vi "RXD_gloval.vi"(7 "종료문자열":string="\r\n", 9 "Vesa_Status":T1=enum."Idel", 11 "SERIAL.COM_Port":refnum<visa-resource-name>="COM1") -> (3 "수신문자":string)   [LabVIEW 2014]
uses:
  VESA_Status.ctl
  bus_button.xctl
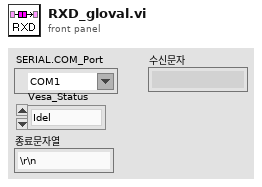
[diagram p1: front panel]
types:
  T1 = typedef "bus_button.xctl/VESA_Status.ctl" = enum16{"Init", "Wait", "Connect", "DisConnect", "Idel", "Exit"}
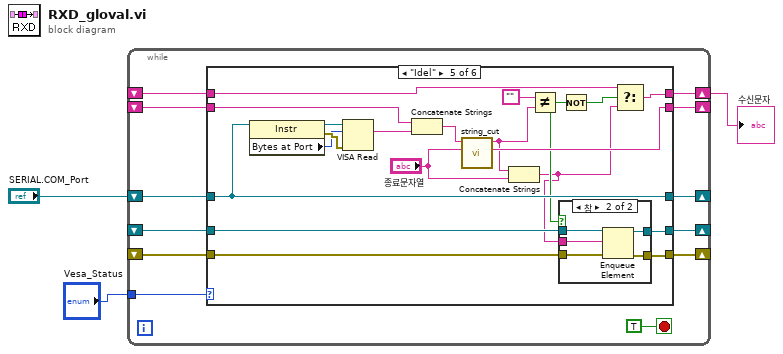
[diagram p0: block diagram]
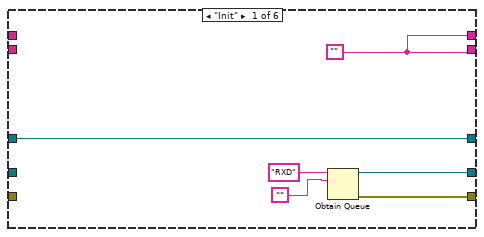
[diagram p2: hidden frame]
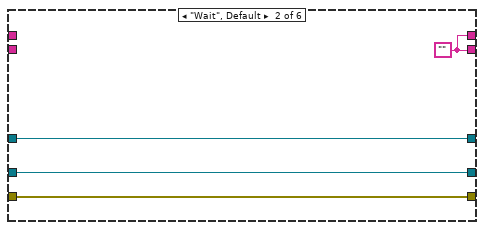
[diagram p3: hidden frame]
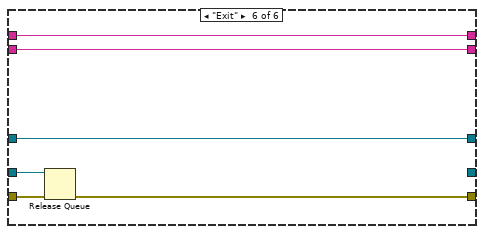
[diagram p7: hidden frame]
diagram:
  n1 = while {
    shift-right: [w14] -> _
    shift-left: _ -> [w10]
    shift-right: [w13] -> _
    shift-left: _ -> [w11]
    shift-right: [w12] -> _
    shift-left: _ -> [w9]
    shift-right: [w7] -> _
    shift-left: "SERIAL.COM_Port" -> [w8]
    tunnel: "Vesa_Status" -> [w6]
    shift-right: [w5] -> w1
    shift-left: _ -> [w4]
    stop <- TRUE stop-if-true
    n2 = case shown="\"Idel\"" w6 {
      tunnel: [w19 w24 w29 w34 w46 _] -> w14
      tunnel: [w18 w25 w30 w35 w47 w64] -> w13
      tunnel: [w16 w22 w28 w33 w43 w68] -> w12
      tunnel: w11 -> [_ w25 w30 w35 w44 w65]
      tunnel: w10 -> [_ w24 w29 w34 w45 w66]
      tunnel: w9 -> [_ _ w28 w33 w51 w68]
      tunnel: w8 -> [w17 w23 w27 w32 w52 w67]
      tunnel: [w17 w23 w27 w32 w52 w67] -> w7
      tunnel: [w16 w22 w26 w31 w41 w63] -> w5
      tunnel: w4 -> [_ _ w26 w31 w39 w63]
      frame "Init" {
        w16 = ""
        n3 = Obtain Queue(name (unnamed)="RXD", element data type="") -> (queue out=w19:refnum<queue>, error out=w18:errorcluster)  [unwired: 3 in, 1 out]
      }
      frame "Wait", Default {
        w22 = ""
      }
      frame "Connect" {
      }
      frame "DisConnect" {
      }
      frame "Idel" {
        n4 = property class="Instr"(reference=w52) -> (reference out=w53:refnum<visa-resource-name>, error out=w55:errorcluster, "Bytes at Port"=w54:u32)  [unwired: 1 in]
        n5 = VISA Read(VISA resource name=w53, byte count=w54, error in (no error)=w55) -> (read buffer=w50:string)  [unwired: 3 out]
        n6 = Concatenate Strings(w51, w50) -> (w49:string)
        n7 = call "string_cut.vi"("종료문자"="종료문자열", "수신문자열"=w49) -> ("나머지문자열"=w43:string, "완성문자열"=w37:string)  [unwired: 7 in, 1 out]
        n8 = Concatenate Strings(w37, "종료문자열") -> (w36:string)
        n9 = Not Equal?(x="", y=w37) -> (x != y?=w42:bool)
        n10 = case shown="참" w42 {
          tunnel: [w56 w62] -> w47
          tunnel: [w57 w61] -> w46
          tunnel: w45 -> [w57 w60]
          tunnel: w44 -> [w56 w59]
          tunnel: w36 -> [_ w58]
          frame False {
          }
          frame True {
            n11 = Enqueue Element(queue=w60, element=w58, error in (no error)=w59) -> (queue out=w61:refnum<queue>, error out=w62:errorcluster)  [unwired: 1 in, 1 out]
          }
        }
        n12 = Not(x=w42) -> (.not. x?=w40:bool)
        n13 = Select(t=w39, s=w40, f=w36) -> (s? t:f=w41:string)
      }
      frame "Exit" {
        n14 = Release Queue(queue=w66, error in (no error)=w65) -> (error out=w64:errorcluster)  [unwired: 1 in, 2 out]
      }
    }
  }
  "수신문자" <- w1
